vi "Table Items.vi"() -> ()   [LabVIEW 2015, in "TDMS datalogger editor node.lvclass"]
uses:
  TDMS datalogger editor node.lvclass
panel:
  in  "Available Tags":string[][](array[string])
  in  "Channels":string[](array[string])
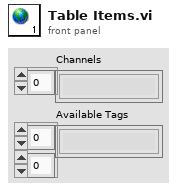
[diagram p1: front panel]
diagram:
